vi "Estacionamiento-VI.vi"() -> (7 "Estacionarse":bool, 8 "Retroceder":bool)   [LabVIEW 2024]
uses:
  Casos estacionamiento.ctl
  Abrir_cerrar pluma.ctl
panel:
  out "Carros en el estacionamiento":i32
  out "Mensaje":string
  in  "Acceso":bool
  in  "Stop Button":bool
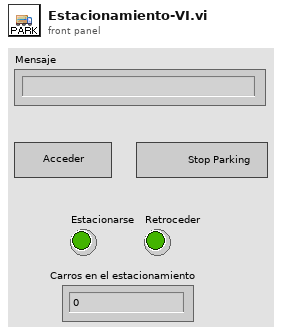
[diagram p1: front panel]
types:
  T1 = typedef "Casos estacionamiento.ctl" = enum16{"Defecto", "Estacionarse", "Retroceder"}
  T2 = typedef "Abrir_cerrar pluma.ctl" = enum16{"Abrir", "Cerrar"}
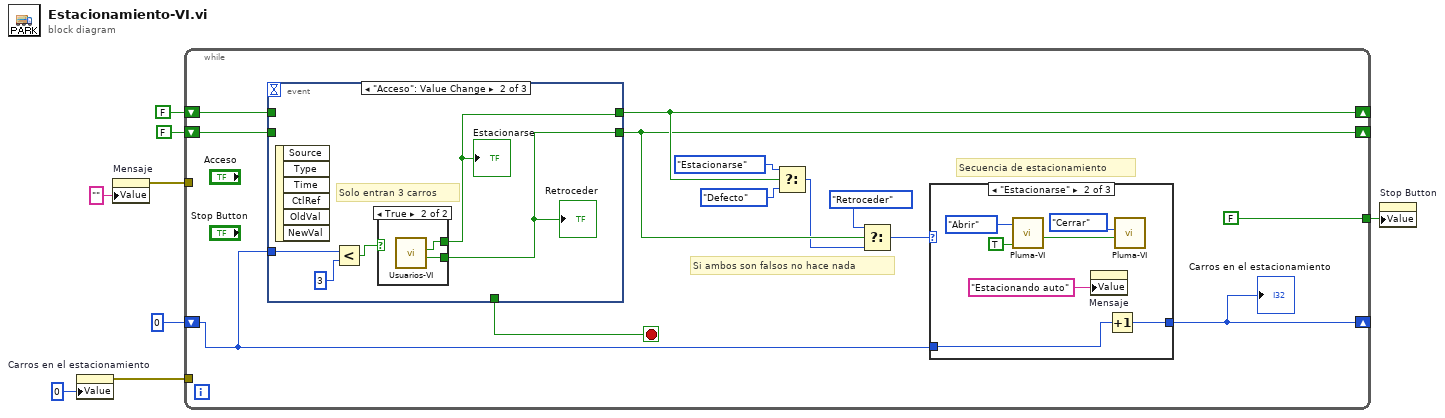
[diagram p0: block diagram]
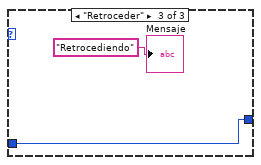
[diagram p3: hidden frame]
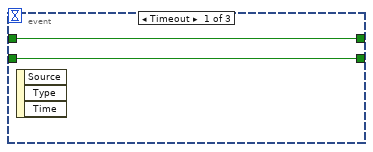
[diagram p4: hidden frame]
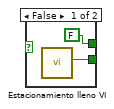
[diagram p5: hidden frame]
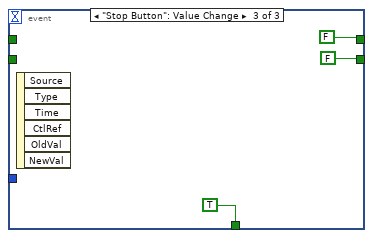
[diagram p6: hidden frame]
diagram:
  n1 = property on="Carros en el estacionamiento" class="DigNum (strict)"("Value"=0 ("Carros en el estacionamiento")) -> (error out=w2:errorcluster)  [unwired: 2 in, 1 out]
  n2 = property on="Mensaje" class="Str"("Value"="" ("Mensaje")) -> (error out=w4:errorcluster)  [unwired: 2 in, 1 out]
  n3 = while {
    tunnel: [FALSE ("Stop Button")] -> w8
    shift-right: [w18] -> _
    shift-left: FALSE ("Estacionarse LED") -> [w19]
    shift-right: [w13] -> _
    shift-left: FALSE ("Retroceder LED") -> [w17]
    shift-right: [w9] -> _
    shift-left: 0 -> [w10]
    tunnel: w4 -> [_]
    tunnel: w2 -> [_]
    stop <- w21 stop-if-true
    # "Si ambos son falsos no hace nada"
    # "Secuencia de estacionamiento"
    n4 = event shown="[1] \"Acceso\": Value Change" {
      selector: _ -> [_ _ _]
      dyn-events: _ -> [_ _ _]
      timeout: _ -> [_ _ _]
      tunnel: [_ _ TRUE] -> w21
      tunnel: [w33 w38 FALSE] -> w18
      tunnel: w19 -> [w33 _ _]
      tunnel: [w32 w37 FALSE] -> w13
      tunnel: w17 -> [w32 _ _]
      tunnel: w10 -> [_ w35 _]
      event Timeout {
        n5 = event-data() -> ()  [unwired: 1 in, 3 out]
      }
      event "Acceso": Value Change {
        # "Solo entran 3 carros"
        n6 = event-data() -> ()  [unwired: 1 in, 6 out]
        n7 = Less?(x=w35, y=3) -> (x < y?=w34:bool)
        n8 = case shown="True" w34 {
          tunnel: [FALSE ("Estacionarse LED") w42] -> w38
          tunnel: [w39 w41] -> w37
          frame False {
            n9 = call "Estacionamiento lleno VI.vi"() -> ("Retroceder LED"=w39:bool)  [unwired: 11 in]
          }
          frame True {
            n10 = call "Usuarios-VI.vi"() -> ("Retroceder LED"=w41:bool, "Estacionarse LED"=w42:bool)  [unwired: 9 in]
          }
        }
        "Retroceder" <- w37
        "Estacionarse" <- w38
      }
      event "Stop Button": Value Change {
        n11 = event-data() -> ()  [unwired: 1 in, 6 out]
      }
    }
    n12 = Select(t=Casos_estacionamiento."Estacionarse", s=w18, f=Casos_estacionamiento."Defecto") -> (s? t:f=w12:T1)
    n13 = Select(t=Casos_estacionamiento."Retroceder", s=w13, f=w12) -> (s? t:f=w11:T1)
    n14 = case shown="\"Estacionarse\"" w11 {
      tunnel: [w22 w24 w30] -> w9
      tunnel: w10 -> [w22 w23 w30]
      frame "Defecto", Default {
      }
      frame "Estacionarse" {
        n15 = call "Pluma-VI.vi"("Parar el funcionamiento"=TRUE, "Pluma"=Abrir_cerrar_pluma."Abrir") -> ("Stop value"=w27:bool)  [unwired: 9 in]
        n16 = property on="Mensaje" class="Str"("Value"="Estacionando auto" ("message")) -> ()  [unwired: 2 in, 2 out]
        n17 = Increment(x=w23) -> (x+1=w24:i32)
        n18 = call "Pluma-VI.vi"("Parar el funcionamiento"=w27, "Pluma"=Abrir_cerrar_pluma."Cerrar") -> ()  [unwired: 9 in, 1 out]
      }
      frame "Retroceder" {
        "Mensaje" <- "Retrocediendo" ("message")
      }
    }
    "Carros en el estacionamiento" <- w9
  }
  n19 = property on="Stop Button" class="Bool (strict)"("Value"=w8) -> ()  [unwired: 2 in, 2 out]
